vi "JSONPath to XPath.vi"(11 "JSONPath":string) -> (3 "XPath":string)   [LabVIEW 2024, in "Config from XML.lvclass"]
uses:
  Config from XML.lvclass
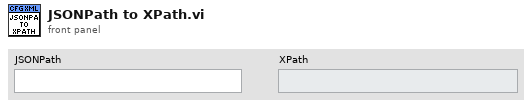
[diagram p1: front panel]
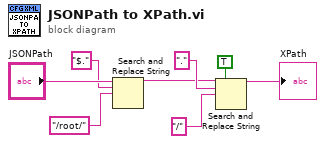
[diagram p0: block diagram]
diagram:
  n1 = Search and Replace String(input string="JSONPath", search string="$.", replace string="/root/" ("replace string (\"\")")) -> (result string=w5:string)  [unwired: 5 in, 3 out]
  n2 = Search and Replace String(replace all?=TRUE ("replace all? (F)"), input string=w5, search string=".", replace string="/" ("replace string (\"\")")) -> (result string=→"XPath":string)  [unwired: 4 in, 3 out]
